vi "Name.vi"(11 "Generic Data Type in":refnum<class "Generic Data Type.lvclass">) -> (2 "String":string="Generic", 3 "Generic Data Type (dup)":refnum<class "Generic Data Type.lvclass">)   [LabVIEW 2018, in "Generic Data Type.lvclass"]
uses:
  Generic Data Type.lvclass
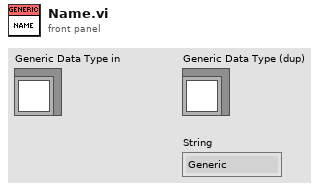
[diagram p1: front panel]
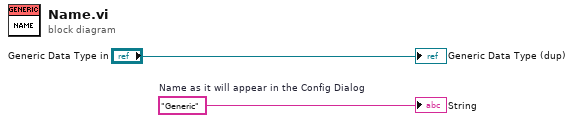
[diagram p0: block diagram]
diagram:
  w1 = "Generic"  # Name as it will appear in the Config Dialog
  "Generic Data Type (dup)" <- "Generic Data Type in"
  "String" <- w1
